vi "Write User Preferences.vi"(8 "error in (no error)":errorcluster, 10 "User Preferences":T1={"Max Recent Experiments"=30.0, "Recent Experiments"=[]}, 11 "User Preferences File in":refnum<class "User Preferences File.lvclass">) -> (0 "error out":errorcluster, 3 "User Preferences File out":refnum<class "User Preferences File.lvclass">)   [LabVIEW 2020, in "User Preferences File.lvclass"]
uses:
  User Preferences File.lvclass
  User Preferences Cluster.ctl
  User Preferences File.lvclass/User Preferences File.ctl
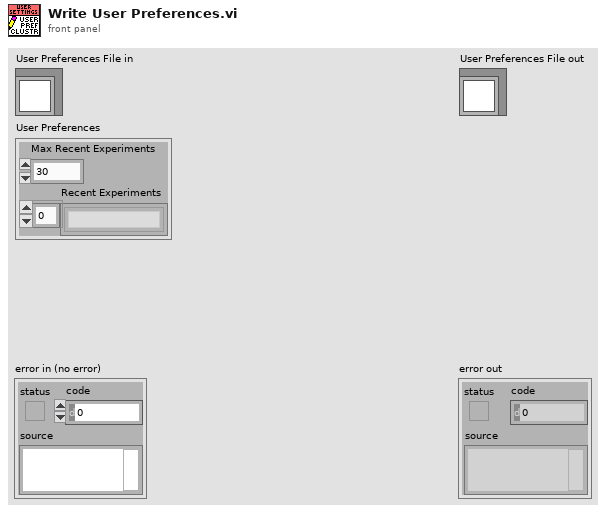
[diagram p1: front panel]
types:
  T1 = typedef "User Preferences File.lvclass/User Preferences Cluster.ctl" = cluster{"Max Recent Experiments":dbl, "Recent Experiments":string[]}
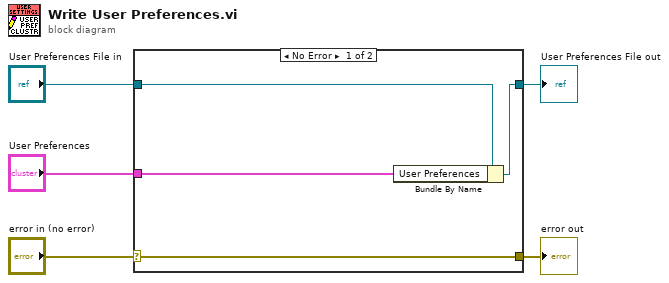
[diagram p0: block diagram]
diagram:
  n1 = case shown="No Error" "error in (no error)" {
    selector: "error in (no error)" -> [w9 w10]
    tunnel: [w9 w10] -> w4
    tunnel: [w7 w11] -> w2
    tunnel: "User Preferences File in" -> [w8 w11]
    tunnel: "User Preferences" -> [w6 _]
    frame No Error {
      n2 = Bundle By Name(cluster=w8, "User Preferences"=w6) -> (w7:refnum<class "User Preferences File.lvclass">)
    }
    frame Error {
    }
  }
  "error out" <- w4
  "User Preferences File out" <- w2
